vi "SMARP Software TCPIP - 100 - TS.vi"() -> (15 "error out":errorcluster={"status"=TRUE, "code"=2, "source"="FT_Open_Device_By_Index_2.vi<ERR>\nFT_DEVICE_NOT_FOUND"})   [LabVIEW 2015]
uses:
  Source code 64 bits/Global Cal Coefficients.vi
  Source code 64 bits/D_MON_Global_Save_Handling.vi
  Source code 64 bits/Global_Trig.vi
  <vilib>/Analysis/NI_AALPro.lvlib
  Source code 64 bits/Global Temp Coefficients.vi
  Source code 64 bits/Global line number.vi
  <vilib>/Utility/file.llb/Write To Spreadsheet File (DBL).vi
panel:
  out "Messages Sent":dbl
  out "String":string
  in  "Wait [ms]":u32=1000
  out "Length":i32
  out "Sending":bool
  in  "Transmission":bool caption="Blank Button"
  out "Scan rate [Hz]":dbl=100.0 format="%.1f"
  out "Total no. of scans":u64=20350
  out "Clear data loss":bool=TRUE
  out "No. of restarts":i16
  out "FT handle":u32=275386408
  in  "Number of pixels":u16=512
  out "Sensor temperature":dbl=29.5
  out "Status":bool=TRUE
  out "No. of scans without \ndata loss":u64=20350
  in  "Dark substraction":enum32{"3", "4"}(radio) caption="Substract dark"
  in  "Default dark spectrum":i32[](array[numeric])
  out "Data loss":bool
  out "Power saturated":bool
  out "Disk streaming enable":bool
  in  "Manuel save\nin datalog file":bool
  out "refnum out":refnum<file>
  out "Fitted Wavelength (nm) 2":dbl[][](array[numeric])=[[1595.5131620083362], [1595.5127751366058], [1595.5137326893469], [1595.5138830332794], [1595.5145223786622], [1595.514016514484], [1595.5136704516492], [1595.5140362639065], [1595.513886981301], [1595.5129422331306], [1595.5142763835854], [1595.5131991204937], [1595.5141702721774], [1595.5140596535118], [1595.513476018252], [1595.5130840632366], [1595.5133372352345], [1595.5143909134829], [1595.512547034042], [1595.5131347474842], [1595.5136018341527], [1595.5133635366617], [1595.5134215597598], [1595.5136216309304], [1595.5134388503177], [1595.514860425136], [1595.513637047946], [1595.5144108307254], [1595.5134006848923], [1595.5136540115332], [1595.5131151127853], [1595.5134841775725], [1595.5135582718326], [1595.51358873526], [1595.5144878935337], [1595.5133866872961], [1595.5135523397537], [1595.513956857277], [1595.5138624036094], [1595.513868537861], [1595.5141773781613], [1595.5139943040829], [1595.5140080784786], [1595.5136054910308], [1595.5132710852274], [1595.5136273367466], [1595.5134180231428], [1595.5137428127452], [1595.5134467206256], [1595.5124864680156], [1595.5133492708483], [1595.5138568551952], [1595.5139521788888], [1595.5129457857986], [1595.5134285012812], [1595.5132775616735], [1595.5138196678542], [1595.5134433791493], [1595.5131057080214], [1595.5135200395807], [1595.513512087234], [1595.512826806178], [1595.5147811740385], [1595.5136915283101], [1595.5137392114034], [1595.5125233078275], [1595.5143754672813], [1595.5137596894583], [1595.5138802243555], [1595.5136627382699], [1595.5128774801633], [1595.512992288448], [1595.5142936144803], [1595.5134010885834], [1595.5132554550344], [1595.5135961940969], [1595.5143572070504], [1595.5132616854469], [1595.5146787806843], [1595.5129005738843], [1595.5139568760248], [1595.5144654170813], [1595.5128774801633], [1595.5132012316803], [1595.5131706301513], [1595.5133248313573], [1595.5142833144234], [1595.5135630852683], [1595.5130317900264], [1595.513331497452], [1595.5139713766837], [1595.5138038514065], [1595.5139041777377], [1595.5136828192435], [1595.5133747159412], [1595.5136313106811], [1595.513910168194], [1595.5137736081301], [1595.5138395201484], [1595.5140244175132], [1595.5143887222805], [1595.513486738009], [1595.5122489667829], [1595.5122830246223], [1595.5131860770355], [1595.5135655715271], [1595.5132986015558], [1595.5129111513875], [1595.513646736944], [1595.512020396329], [1595.5133269476487], [1595.513158439359], [1595.5133154608318], [1595.513528581914], [1595.514587517312], [1595.513215473403], [1595.5133411671345], [1595.512850376517], [1595.513826716082], [1595.513113875053], [1595.5140448881584], [1595.5138417196122], [1595.5127217640932], [1595.5137354831563], [1595.5134230825417], [1595.5135733593886], [1595.2929746856532], [1595.51298986152], [1595.513021410847], [1595.5131545750744]] format="%.3f"
  out "Power Array":dbl[][](array[numeric]) format="%.2f"
  out "Dark spectrum":dbl[](array[numeric])
  in  "origin 2":cluster{"x":i16, "y":i16}
  out "new picture 2":picture
  in  "origin":cluster{"x":i16, "y":i16}={"x"=0, "y"=10}
  out "Fitted Wavelength (nm)":dbl[][](array[numeric]) format="%.4f"
  in  "Tab Control":T1(tab)
  out "Spectrum  Graph":cluster{dbl[], "Line spectrums":dbl[]}(graph)
  in  "Exposure time [usec]":dbl=10000.0 min=3.0 max=65535.0
  out "Wavelength Graph":T2(graph)={"f"=0.0, 0.0003333333333333333, "Rearranged array"=[]}
  out "Peak Frequency [Hz]":dbl[][](array[numeric]) format="%.2f"
  in  "FFT peak threshold [nm]":dbl=0.0005999999999999925 min=0.0 step=0.0001 format="%.5f"
  out "FFT Graph":T3(graph)
  in  "FFT calculation":enum32{"pix", "nm"}(radio)
  in  "Change datalog\nfile name":bool
  in  "Timed  data log":bool
  in  "Raw data collection":enum32{"3", "4"}(radio)
  in  "Disc streaming":enum32{"1", "2"}(radio)
  in  "X-Axis unit":enum32{"pix", "nm"}(radio)=enum."nm"
  in  "Measurement trig type":enum16{"Manuel", "Auto", "Continuous"}(ring)=enum."Continuous"
  in  "Max number \nof FBG's":u16=20 min=1
  in  "Threshold [%]":dbl=10.0
  in  "No. of frames to disc unified":i32=100
  in  "Trig frequency [Hz]":dbl=0.5 format="%.2f"
  in  "Circular Sample \nbuffer length":i32=3000
  in  "Wavelength/FFT graph buffer length":i32=3000
  out "Calibration coefficients":dbl[](array[numeric])=[1595.998689, -0.1387869764, -6.248194306e-05, -3.744159492e-09, 6.889567755e-13, -1.540737e-15] format="%.6e"
  out "Temperature coefficients":dbl[](array[numeric])=[-1.034429555e-06, 3.155140097e-05, -0.0001139713184, -0.004721861303] format="%.6e"
  in  "Change Disk stream\nfile name":bool
  in  "Neighbours in fit":i32=1
  in  "Change datalog\ntime interval":bool
  in  "Temperature \ncompensation":bool=TRUE
  in  "Exposure time\n[usec]":dbl=10000.0 min=3.0 max=65535.0
  in  "Fit Type":enum32{"Gauss", "COG", "COG DWA", "No fit"}(radio)=enum."COG DWA"
  in  "Max Scan rate [Hz]":i32=100 min=1 max=3000
  in  "No. of lines \nunified":u16=10 min=1 max=100 step=1
  in  "Offset (-250..250) mV":i32=-88
  in  "Path":path
  in  "Save Raw":bool
  in  "Save Wave":bool
  in  "Trig":bool
  in  "Exit":bool
  # "Ver 1.3"
  # "Peak no."
  # "Sample no."
  # "Peak no."
  # "FFT peak"
  # "Buffer setup"
  # "Camera setup"
  # "File setup"
  # "Interrogation setup"
  # "SW Trig setup"
  # "ID  information"
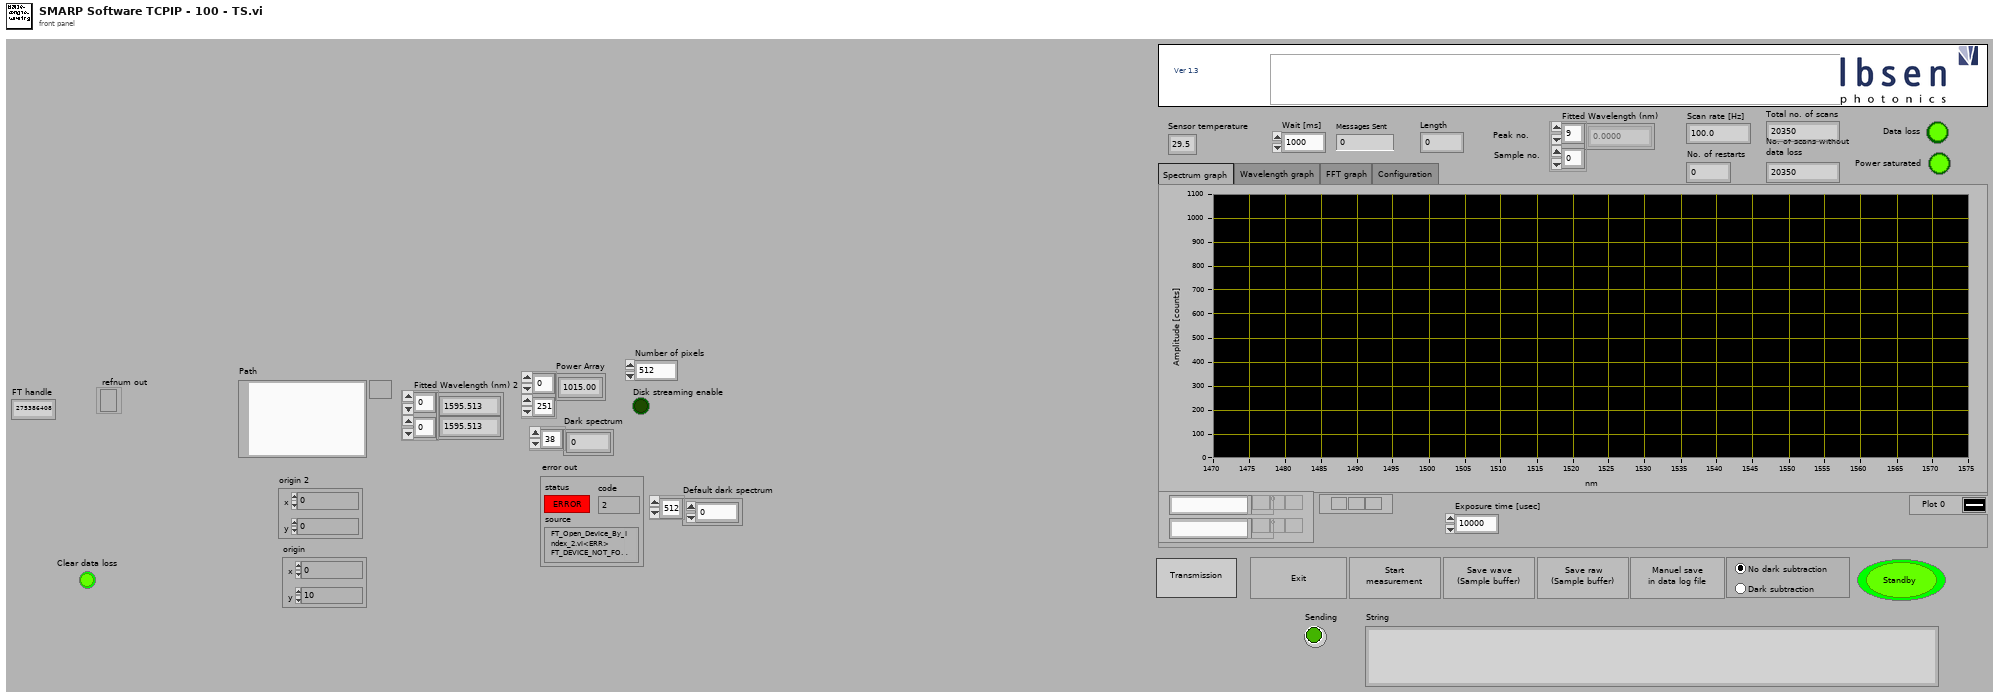
[diagram p1: front panel]
types:
  T1 = enum32{"Spectrum graph", "Wavelength graph", "FFT graph", "Configuration"}
  T2 = cluster{"f":dbl, dbl, "Rearranged array":dbl[][]}
  T3 = cluster{dbl, "df":dbl, "Amp Spectrum Mag (Vrms)":dbl[][]}
  T4 = enum16{"User-specified Font", "Application Font", "System Font", "Dialog Font"}
  T5 = cluster{"Font Name:":string, "Size":i16, "Strikeout?":bool, "Italic?":bool, "Underline?":bool, "Outline?":bool, "Shadow?":bool, "Bold?":bool}
  T6 = enum16{"open", "replace", "create", "open or create", "replace or create", "replace or create with confirmation"}
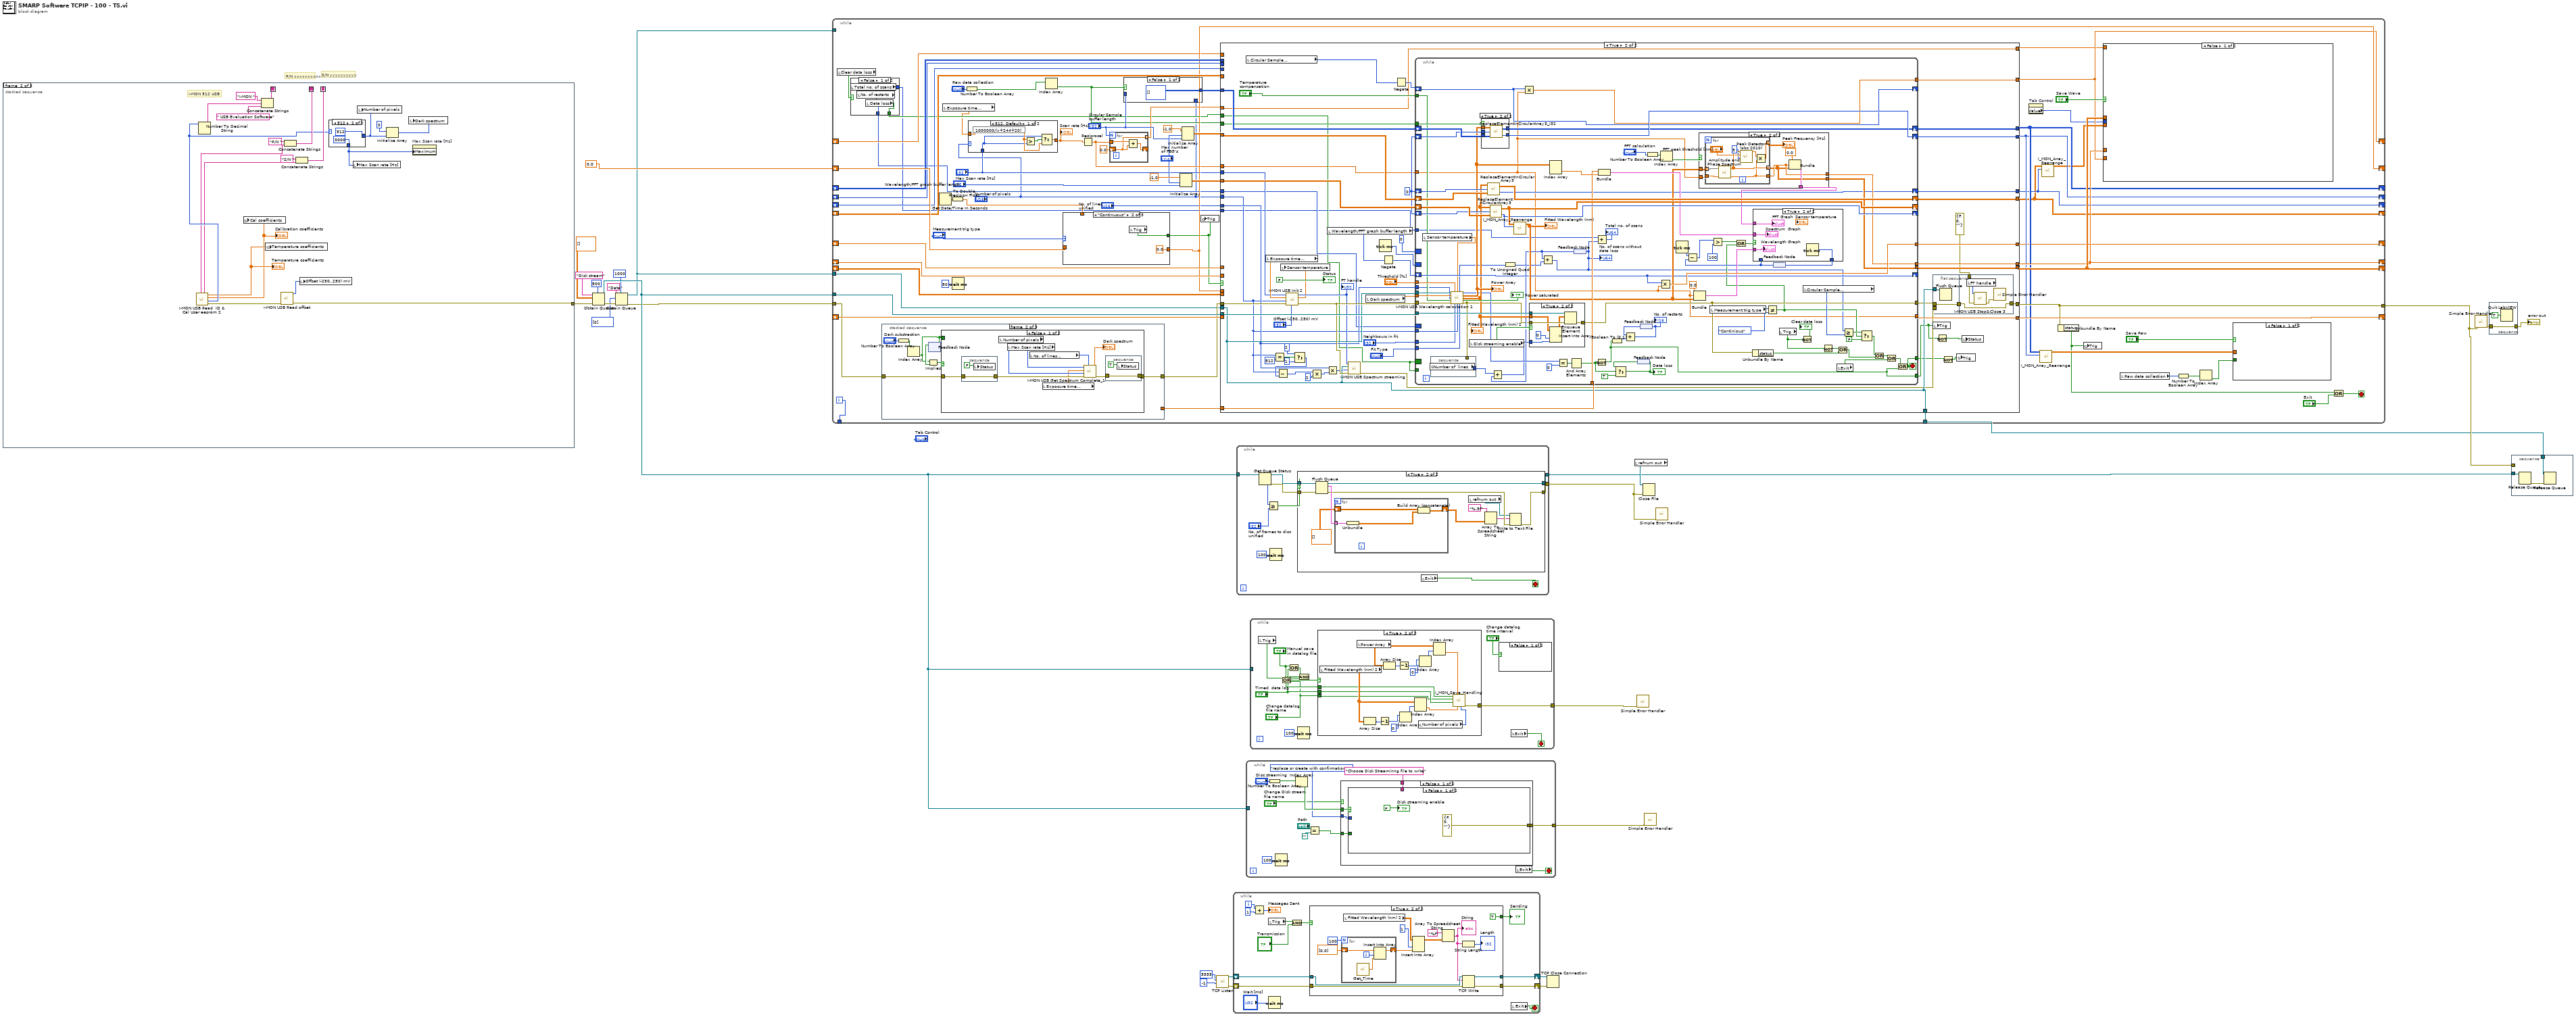
[diagram p0: block diagram]
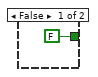
[diagram p2: hidden frame]
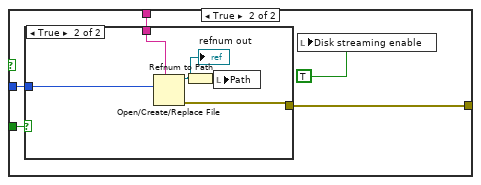
[diagram p3: hidden frame]
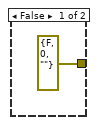
[diagram p4: hidden frame]
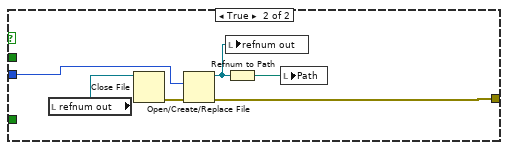
[diagram p5: hidden frame]
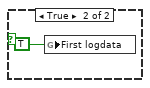
[diagram p6: hidden frame]
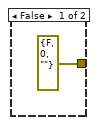
[diagram p7: hidden frame]
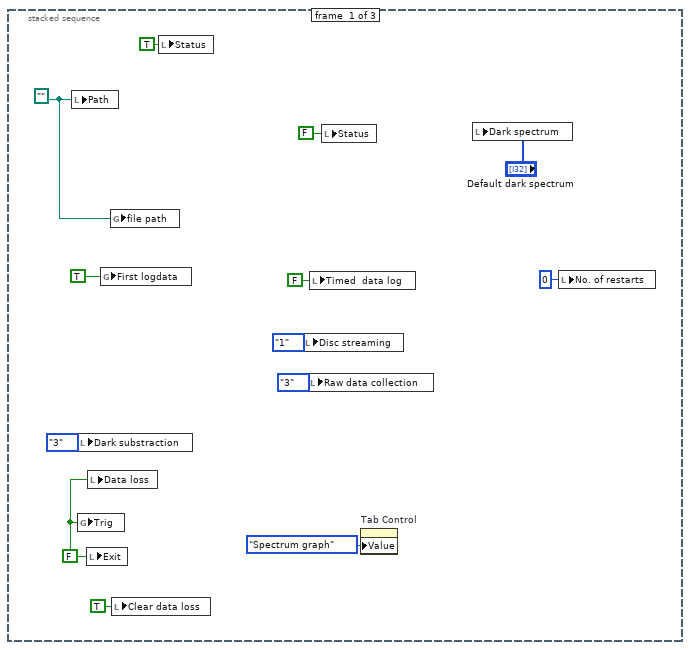
[diagram p8: hidden frame]
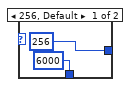
[diagram p9: hidden frame]
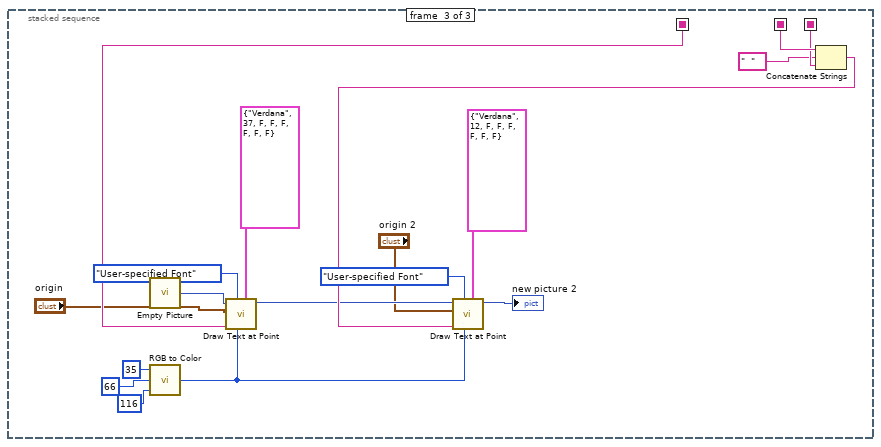
[diagram p10: hidden frame]
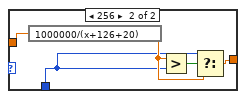
[diagram p12: hidden frame]
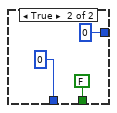
[diagram p13: hidden frame]
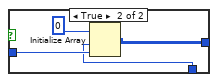
[diagram p14: hidden frame]
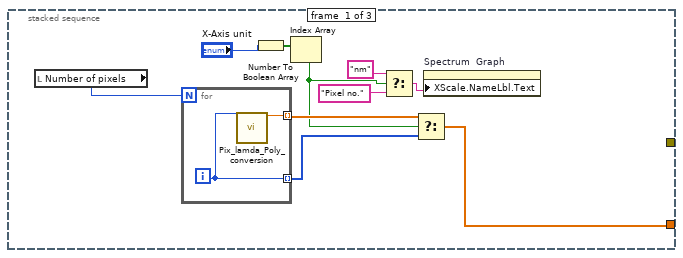
[diagram p15: hidden frame]
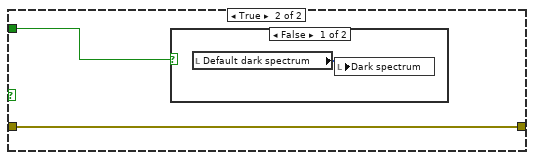
[diagram p16: hidden frame]
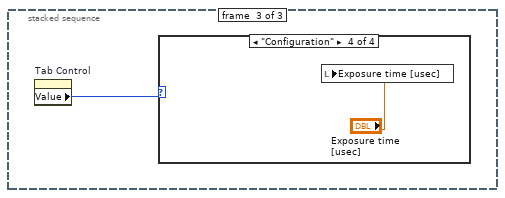
[diagram p18: hidden frame]
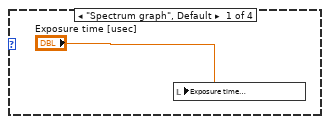
[diagram p19: hidden frame]
diagram:
  # "S/N yyyyyyyyyy"
  # "P/N xxxxxxxxxx"
  n1 = stacked-sequence {
    seq-local: [_ w60 _] -> [_ _ w71]
    seq-local: [_ w59 _] -> [_ _ w66]
    seq-local: [_ w57 _] -> [_ _ w76]
    tunnel: [_ w43 _] -> w22
    frame #0 {
      w29 = FALSE ("Exit")
      w37 = path ""
      n2 = local write "Path"(w37) -> ()
      n3 = local write "Dark substraction"(enum32{"3", "4"}."3" ("Dark substraction")) -> ()
      n4 = global write "Global_Trig.vi" "Trig"(w29) -> ()
      n5 = local write "Exit"(w29) -> ()
      n6 = local write "Data loss"(w29) -> ()
      n7 = global write "D_MON_Global_Save_Handling.vi" "First logdata"(TRUE ("First logdata")) -> ()
      n8 = global write "D_MON_Global_Save_Handling.vi" "file path"(w37) -> ()
      n9 = local write "Clear data loss"(TRUE ("Clear data loss")) -> ()
      n10 = local write "Status"(TRUE ("OK")) -> ()
      n11 = local write "Disc streaming"(enum32{"1", "2"}."1" ("Disk streaming")) -> ()
      n12 = local write "Raw data collection"(enum32{"3", "4"}."3" ("Raw data collection")) -> ()
      n13 = local write "Timed  data log"(FALSE ("Timed  datalog")) -> ()
      n14 = local write "Status"(FALSE ("Status")) -> ()
      n15 = property on="Tab Control" class="TabCtl (strict)"("Value"=T1."Spectrum graph" ("Tab Control")) -> ()  [unwired: 2 in, 2 out]
      n16 = local write "Dark spectrum"("Default dark spectrum") -> ()
      n17 = local write "No. of restarts"(i16 0 ("No. of restarts")) -> ()
    }
    frame #1 {
      # "I-MON 512 USB"
      n18 = call "I-MON USB Read  ID & Cal User eeprom 2.vi"() -> ("error out"=w44:errorcluster, "No. of pixels"=w51:i32, "Wave Cal coef"=w45:dbl[], "Temp Cal coef"=w46:dbl[], "Serial no."=w47:string, "Part no."=w49:string)  [unwired: 6 in]
      "Calibration coefficients" <- w45
      "Temperature coefficients" <- w46
      n19 = Number To Decimal String(number=w51) -> (decimal integer string=w52:string)  [unwired: 1 in]
      n20 = global write "Global Cal Coefficients.vi" "Cal coefficients"(w45) -> ()
      n21 = Concatenate Strings("I-MON " ("string"), w52, " USB Evaluation Software" ("text")) -> (w57:string)
      n22 = global write "Global Temp Coefficients.vi" "Temperature coefficients"(w46) -> ()
      n23 = call "I-MON USB Read offset.vi"("error in (no error)"=w44) -> ("error out"=w43:errorcluster, "Offset"=w42:i32)  [unwired: 9 in]
      n24 = Concatenate Strings("P/N " ("string"), w49) -> (w60:string)
      n25 = Concatenate Strings("S/N " ("string"), w47) -> (w59:string)
      n26 = local write "Offset (-250..250) mV"(w42) -> ()
      n27 = case shown="512" w51 {
        tunnel: [256 ("CCD Type") 512 ("CCD Type")] -> w55
        tunnel: [6000 ("CCD Type") 3000 ("CCD Type")] -> w41
        frame 256, Default {
        }
        frame 512 {
        }
      }
      n28 = local write "Max Scan rate [Hz]"(w41) -> ()
      n29 = local write "Number of pixels"(w55) -> ()
      n30 = Initialize Array(0, w55) -> (w54:i32[])
      n31 = local write "Dark spectrum"(w54) -> ()
      n32 = property on="Max Scan rate [Hz]" class="DigNum (strict)"("Maximum"=w41) -> ()  [unwired: 2 in, 2 out]
    }
    frame #2 {
      n33 = call "Empty Picture"() -> ("empty picture"=w82:picture)
      n34 = call <vilib>:"RGB to Color.vi"("B"=u8 116, "G"=u8 66, "R"=u8 35) -> ("Color"=w73:u32)
      n35 = call <vilib>:"Draw Text at Point.vi"("[user-specified font]"=T5 {"Font Name:"="Verdana", "Size"=37, "Strikeout?"=FALSE, "Italic?"=FALSE, "Underline?"=FALSE, "Outline?"=FALSE, "Shadow?"=FALSE, "Bold?"=FALSE}, "text color(black)"=w73, "desired font(Application)"=T4."User-specified Font", "text"=w76, "origin"="origin", "picture"=w82) -> ("new picture"=w68:picture)  [unwired: 4 in, 1 out]
      n36 = Concatenate Strings(w71, "  " ("string"), w66) -> (w70:string)
      n37 = call <vilib>:"Draw Text at Point.vi"("[user-specified font]"=T5 {"Font Name:"="Verdana", "Size"=12, "Strikeout?"=FALSE, "Italic?"=FALSE, "Underline?"=FALSE, "Outline?"=FALSE, "Shadow?"=FALSE, "Bold?"=FALSE}, "text color(black)"=w73, "desired font(Application)"=T4."User-specified Font", "text"=w70, "origin"="origin 2", "picture"=w68) -> ("new picture"=→"new picture 2":picture)  [unwired: 4 in, 1 out]
    }
  }
  n38 = Obtain Queue(max queue size (-1, unlimited)=500, name (unnamed)="Disk stream", element data type=dbl[][] [], error in (no error)=w22) -> (queue out=w18:refnum<queue>, error out=w16:errorcluster)  [unwired: 1 in, 1 out]
  n39 = Obtain Queue(max queue size (-1, unlimited)=1000, name (unnamed)="Data", element data type=u8[] [0], error in (no error)=w16) -> (queue out=w11:refnum<queue>, error out=w15:errorcluster)  [unwired: 1 in, 1 out]
  n40 = while {
    tunnel: [w134] -> w23
    shift-right: [w117] -> _
    shift-left: 0.0 ("seconds since 1Jan1904") -> [w147]
    shift-right: [w143] -> _
    shift-left: _ -> [w144]
    shift-right: [w142] -> _
    shift-left: _ -> [w140]
    shift-right: [w139] -> _
    shift-left: _ -> [w141]
    tunnel: w15 -> [w109]
    shift-right: [w121] -> _
    shift-left: _ -> [w129]
    shift-right: [w122] -> _
    shift-left: _ -> [w128]
    shift-right: [w123] -> _
    shift-left: _ -> [w125]
    shift-right: [w124] -> _
    shift-left: _ -> [w126]
    shift-right: [w118] -> _
    shift-left: _ -> [w119]
    shift-right: [w115] -> _
    shift-left: _ -> [w116]
    tunnel: w18 -> [w114]
    tunnel: w11 -> [_]
    tunnel: w11 -> [w106]
    tunnel: [w105] -> w10
    tunnel: [w103] -> _
    i -> [w103]
    stop <- w149 stop-if-true
    n41 = local read "Clear data loss"() -> (w91:bool)
    n42 = case shown="False" w91 {
      tunnel: [w163 i16 0] -> w93
      tunnel: [w162 FALSE ("Data loss")] -> w92
      tunnel: [w161 u64 0 ("Total no. of scans")] -> w90
      frame False {
        n43 = local read "Total no. of scans"() -> (w161:u64)
        n44 = local read "No. of restarts"() -> (w163:i16)
        n45 = local read "Data loss"() -> (w162:bool)
      }
      frame True {
      }
    }
    n46 = stacked-sequence {
      tunnel: [w182 _ _] -> w112
      tunnel: w109 -> [_ w193 _]
      tunnel: [_ w192 _] -> w108
      frame #0 {
        n47 = local read "Number of pixels"() -> (w175:u16)
        n48 = for {
          N: w175 -> [_]
          tunnel: [w186] -> w183 mode=indexing
          tunnel: [w185] -> w184 mode=indexing
          i -> [w185]
          n49 = call "Pix_lamda_Poly_conversion.vi"("Pixels"=w185) -> ("Lamda(nm)"=w186:dbl)  [unwired: 8 in, 6 out]
        }
        n50 = Number To Boolean Array(number="X-Axis unit") -> (Boolean array=w181:bool[])
        n51 = Index Array(array=w181) -> (element=w176:bool)  [unwired: 1 in]
        n52 = Select(t="nm", s=w176, f="Pixel no.") -> (s? t:f=w179:string)
        n53 = Select(t=w183, s=w176, f=w184) -> (s? t:f=w182:dbl[])
        n54 = property on="Spectrum  Graph" class="XYGraph (strict)"("XScale.NameLbl.Text"=w179) -> ()  [unwired: 2 in, 2 out]
      }
      frame #1 {
        n55 = Number To Boolean Array(number="Dark substraction") -> (Boolean array=w189:bool[])
        n56 = Index Array(array=w189) -> (element=w187:bool)  [unwired: 1 in]
        n57 = feedback-in #1(w187) -> ()
        n58 = feedback #1() -> (w191:bool)  [unwired: 1 in]
        n59 = Implies(1:w191, 2:w187) -> (0:w190:bool)
        n60 = case shown="False" w190 {
          tunnel: w193 -> [w202 w208]
          tunnel: [w200 w208] -> w192
          tunnel: w187 -> [_ w207]
          frame False {
            n61 = stacked-sequence {
              tunnel: w202 -> [w205]
              tunnel: [w205] -> w201
              frame #0 {
                n62 = local write "Status"(FALSE ("Status")) -> ()
              }
            }
            n63 = local read "Number of pixels"() -> (w195:u16)
            n64 = local read "Max Scan rate [Hz]"() -> (w196:i32)
            n65 = local read "No. of lines \nunified"() -> (w197:u16)
            n66 = local read "Exposure time\n[usec]"() -> (w194:dbl)
            n67 = call "I-MON USB Get Spectrum Complete_1.vi"("Number of avg spectrums"=w197, "error in (no error)"=w201, "No of pixels"=w195, "Integration time [us]"=w194, "Sample frequency"=w196) -> ("error out"=w198:errorcluster, "Line spectrums"=→"Dark spectrum":dbl[])  [unwired: 5 in]
            n68 = stacked-sequence {
              tunnel: w198 -> [w203]
              tunnel: [w203] -> w200
              frame #0 {
                n69 = local write "Status"(TRUE ("Status")) -> ()
              }
            }
          }
          frame True {
            n70 = case shown="False" w207 {
              frame False {
                n71 = local read "Default dark spectrum"() -> (w209:i32[])
                n72 = local write "Dark spectrum"(w209) -> ()
              }
              frame True {
              }
            }
          }
        }
      }
      frame #2 {
        n73 = property on="Tab Control" class="TabCtl (strict)"() -> ("Value"=w210:T1)  [unwired: 2 in, 2 out]
        n74 = case shown="\"Configuration\"" w210 {
          frame "Spectrum graph", Default {
            n75 = local write "Exposure time\n[usec]"("Exposure time [usec]") -> ()
          }
          frame "Wavelength graph" {
          }
          frame "FFT graph" {
          }
          frame "Configuration" {
            n76 = local write "Exposure time [usec]"("Exposure time\n[usec]") -> ()
          }
        }
      }
    }
    n77 = Get Date/Time In Seconds() -> (seconds since 1Jan1904=w138:timestamp)
    n78 = local read "Exposure time\n[usec]"() -> (w86:dbl)
    n79 = To Double Precision Float(number=w138) -> (double precision float=w148:dbl)
    n80 = Wait (ms)(milliseconds to wait=u32 50) -> ()  [unwired: 1 out]
    n81 = Number To Boolean Array(number="Raw data collection") -> (Boolean array=w110:bool[])
    n82 = case shown="512, Default" "Number of pixels" {
      tunnel: w86 -> [w153 w160]
      tunnel: [w152 w157] -> w83
      tunnel: "Max Scan rate [Hz]" -> [w151 w156]
      frame 512, Default {
        n83 = expression code="1000000/(x+244+20)"(w153) -> (w154:dbl)
        n84 = Greater?(x=w154, y=w151) -> (0:w155:bool)
        n85 = Select(t=w151, s=w155, f=w154) -> (s? t:f=w152:dbl)
      }
      frame 256 {
        n86 = expression code="1000000/(x+126+20)"(w160) -> (w158:dbl)
        n87 = Greater?(x=w158, y=w156) -> (0:w159:bool)
        n88 = Select(t=w156, s=w159, f=w158) -> (s? t:f=w157:dbl)
      }
    }
    "Scan rate [Hz]" <- w83
    n89 = Index Array(array=w110) -> (element=w89:bool)  [unwired: 1 in]
    n90 = case shown="\"Continuous\"" "Measurement trig type" {
      tunnel: w148 -> [_ _ w285]
      tunnel: [0.0 ("seconds since 1Jan1904") 0.0 ("seconds since 1Jan1904") w283] -> w117
      tunnel: w147 -> [_ _ w278]
      tunnel: ["Trig" w277 w280] -> w104
      frame "Manuel", Default {
      }
      frame "Continuous" {
        n91 = local read "Trig"() -> (w277:bool)
      }
      frame "Auto" {
        n92 = Reciprocal(x="Trig frequency [Hz]") -> (1/x=w281:dbl)
        n93 = Add(x=w278, y=w281) -> (x+y=w279:dbl)
        n94 = Greater Or Equal?(x=w285, y=w279) -> (x >= y?=w284:bool)
        n95 = case shown="False" w284 {
          tunnel: [w287 w290] -> w283
          tunnel: w278 -> [w287 _]
          tunnel: [w286 w288] -> w280
          frame False {
            w286 = FALSE
            n96 = local write "Trig"(w286) -> ()
          }
          frame True {
            w288 = TRUE
            n97 = Get Date/Time In Seconds() -> (seconds since 1Jan1904=w289:timestamp)
            n98 = local write "Trig"(w288) -> ()
            n99 = To Double Precision Float(number=w289) -> (double precision float=w290:dbl)
          }
        }
      }
    }
    n100 = Reciprocal(x=w83) -> (1/x=w87:dbl)
    n101 = for {
      N: "Circular Sample \nbuffer length" -> [_]
      tunnel: w87 -> [w168]
      shift-right: [w169] -> _
      shift-left: 0.0 -> [w167]
      tunnel: [w167] -> w95 mode=indexing
      n102 = Add(x=w168, y=w167) -> (x+y=w169:dbl)
    }
    n103 = case shown="False" w89 {
      tunnel: "Circular Sample \nbuffer length" -> [_ w174]
      tunnel: [i32[][] [] ("f") w172] -> w107
      tunnel: "Number of pixels" -> [_ w171]
      frame False {
      }
      frame True {
        n104 = Initialize Array(u16 0, w171, w174) -> (w172:u16[][])
      }
    }
    n105 = Initialize Array(-1.0 ("element"), "Max number \nof FBG's", "Wavelength/FFT graph buffer length") -> (w131:dbl[][])
    n106 = Initialize Array(-1.0 ("element"), "Max number \nof FBG's", "Circular Sample \nbuffer length") -> (w135:dbl[][])
    n107 = global write "Global_Trig.vi" "Trig"(w104) -> ()
    n108 = case shown="True" w104 {
      tunnel: [w292 w341] -> w134
      tunnel: w117 -> [_ _]
      tunnel: [w302 w363] -> w143
      tunnel: w144 -> [w302 _]
      tunnel: [w300 w362] -> w142
      tunnel: [w301 w360] -> w139
      tunnel: w141 -> [w301 _]
      tunnel: w140 -> [w300 _]
      tunnel: w108 -> [w292 w361]
      tunnel: w135 -> [_ w359]
      tunnel: w131 -> [_ w358]
      tunnel: [w299 w355] -> w121
      tunnel: [w298 w354] -> w122
      tunnel: w129 -> [w299 _]
      tunnel: w128 -> [w298 _]
      tunnel: w107 -> [_ w353]
      tunnel: [w297 w352] -> w124
      tunnel: [w296 w351] -> w123
      tunnel: w126 -> [w297 _]
      tunnel: w125 -> [w296 _]
      tunnel: [w295 w350] -> w118
      tunnel: w119 -> [w295 _]
      tunnel: [w294 w348] -> w115
      tunnel: w116 -> [w294 _]
      tunnel: w89 -> [_ w346]
      tunnel: w114 -> [_ w345]
      tunnel: w112 -> [_ w344]
      tunnel: w106 -> [w293 w333]
      tunnel: [w293 w333] -> w105
      tunnel: "Max Scan rate [Hz]" -> [_ w327]
      tunnel: "No. of lines \nunified" -> [_ w314]
      tunnel: "Number of pixels" -> [_ w313]
      tunnel: w95 -> [w291 w311]
      tunnel: [w291 w311] -> w94
      tunnel: w93 -> [_ w309]
      tunnel: w92 -> [_ w308]
      tunnel: w90 -> [_ w305]
      tunnel: w87 -> [_ w303]
      frame False {
      }
      frame True {
        w338 = u32 0
        n109 = local read "Circular Sample \nbuffer length"() -> (w336:i32)
        n110 = local read "Exposure time\n[usec]"() -> (w328:dbl)
        n111 = Equal?(x=w313, y=u16 512) -> (x = y?=w321:bool)
        n112 = call "I-MON USB Init 2.vi"("Offset (-250..250) mV"="Offset (-250..250) mV", "error in (no error)"=w361, "No of pixels"=w313, "Integration time [us]"=w328, "Max Sample frequency"=w327) -> ("error out"=w340:errorcluster, "Temperature"=w312:dbl, "Handle"=w323:u32)  [unwired: 4 in]
        "FT handle" <- w323
        n113 = local write "Sensor temperature"(w312) -> ()
        n114 = Select(t=u16 2 ("y"), s=w321, f=u16 1) -> (s? t:f=w317:u16)
        n115 = Subtract(x=w313, y=w317) -> (x-y=w316:u16)
        n116 = Multiply(x=w316, y=2) -> (x*y=w324:i32)
        n117 = Multiply(x=w314, y=w324) -> (x*y=w318:i32)
        n118 = local read "Wavelength/FFT graph buffer length"() -> (w337:i32)
        n119 = call "I-MON USB Spectrum streaming.vi"("error in (no error)"=w340, "Bytes To Read"=w318, "queue in"=w333, "Handle"=w323) -> ("error out"=w331:errorcluster)  [unwired: 7 in]
        n120 = local read "Dark spectrum"() -> (w343:dbl[])
        n121 = Tick Count (ms)() -> (millisecond timer value=w342:u32)
        n122 = Negate(x=w337) -> (-x=w357:i32)
        n123 = Negate(x=w336) -> (-x=w349:i32)
        n124 = while {
          tunnel: w340 -> [w458]
          tunnel: [w429] -> w332
          tunnel: [w414] -> w363
          tunnel: [w415] -> w362
          tunnel: "Fit Type" -> [w399]
          tunnel: [w370] -> w360
          shift-right: [w409] -> w354
          shift-left: w338 -> [w455]
          shift-right: [w453] -> w355
          shift-left: w359 -> [w454]
          shift-right: [w437] -> _
          shift-left: w358 -> [w456]
          shift-right: [w436] -> _
          shift-left: w338 -> [w452]
          shift-right: [w412] -> _
          shift-left: w357 -> [w412]
          shift-right: [w438] -> w352
          shift-left: w353 -> [w444]
          shift-right: [w443] -> w351
          shift-left: w338 -> [w442]
          tunnel: [w441] -> w350
          shift-right: [w411] -> _
          shift-left: w349 -> [w411]
          tunnel: [w440] -> w348
          tunnel: "Threshold [%]" -> [w439]
          tunnel: w303 -> [w370]
          border: w308 -> [_]
          tunnel: w346 -> [w435]
          tunnel: w345 -> [w434]
          tunnel: w344 -> [w432]
          tunnel: w343 -> [w405]
          tunnel: w333 -> [w406]
          border: w342 -> [_]
          tunnel: "Temperature \ncompensation" -> [w404]
          tunnel: w313 -> [w398]
          tunnel: "Neighbours in fit" -> [w397]
          tunnel: w314 -> [w396]
          tunnel: w308 -> [_]
          border: u64 0 -> [_]
          tunnel: [w387] -> w310
          border: w309 -> [_]
          tunnel: [w382] -> w307
          tunnel: w305 -> [w378]
          stop <- w382 stop-if-true
          n125 = local read "Sensor temperature"() -> (w403:dbl)
          n126 = call "I-MON USB Wavelength calculation 1.vi"("queue"=w406, "Threshold\n[%]"=w439, "PCB temperature"=w403, "Dark meas"=w405, "No. of spectrums"=w396, "Temp. compensation"=w404, "error in (no error)"=w458, "Neighbours in fit"=w397, "Number of pixels"=w398, "Fit Type"=w399) -> ("No. of line scans"=w391:i32, "Delimiter"=w394:u16[], "Line spectrums"=w401:dbl[][], "Center pixels (0 indexeret)"=w400:dbl[][], "Power saturated"=→"Power saturated":bool, "error out"=w372:errorcluster)
          "Power Array" <- w401
          "Fitted Wavelength (nm) 2" <- w400
          n127 = stacked-sequence {
            tunnel: [w459] -> w375
            tunnel: w372 -> [_]
            frame #0 {
              n128 = global read "Global line number.vi" "Number of  lines"() -> (w459:i32[])
            }
          }
          n129 = local read "Disk streaming enable"() -> (w433:bool)
          n130 = case shown="True" w435 {
            tunnel: w401 -> [_ w497]
            tunnel: w444 -> [w492 w496]
            tunnel: [w491 w495] -> w443
            tunnel: w442 -> [w491 w494]
            tunnel: [w492 w493] -> w438
            frame False {
            }
            frame True {
              n131 = call "ReplaceElementInCircularArray3_I32.vi"("Initial Array - Before Element Inserted"=w496, "Original Element's Index"=w494, "Inserted Array"=w497) -> ("New Element Index \nfor Circular Array"=w495:u32, "Output Circular Array - After Inserting Element"=w493:i32[][])
            }
          }
          n132 = call "ReplaceElementInCircularArray3.vi"("Initial Array - Before Element Inserted"=w454, "Original Element's Index"=w455, "Inserted Array"=w400) -> ("New Element Index \nfor Circular Array"=w409:u32, "Output Circular Array - After Inserting Element"=w453:dbl[][])
          n133 = call "ReplaceElementInCircularArray3.vi"("Initial Array - Before Element Inserted"=w456, "Original Element's Index"=w452, "Inserted Array"=w400) -> ("New Element Index \nfor Circular Array"=w436:u32, "Output Circular Array - After Inserting Element"=w437:dbl[][])
          n134 = To Unsigned Quad Integer(1:w391) -> (0:w377:u64)
          n135 = call "I_MON_Array_Rearrange.vi"("index"=w436, "Initial Array"=w437) -> ("Rearranged array"=w416:dbl[][])  [unwired: 9 in]
          "Fitted Wavelength (nm)" <- w416
          n136 = Multiply(x=w411, y=w370) -> (x*y=w440:dbl)
          n137 = Index Array(array=w401) -> (element=w431:dbl[])  [unwired: 2 in]
          n138 = Equal?(x=w394, y=u16 0 ("Delimiter")) -> (x = y?=w395:bool[])
          n139 = And Array Elements(Boolean array=w395) -> (logical AND=w390:bool)
          n140 = feedback #2() -> (w373:u64)
          n141 = Add(x=w375, y=w373) -> (x+y=w374:u64[])
          n142 = case shown="True" w433 {
            tunnel: w434 -> [_ w490]
            tunnel: w400 -> [_ w486]
            tunnel: w372 -> [w483 w489]
            tunnel: [w483 w488] -> w429
            tunnel: w374 -> [_ w484]
            frame False {
            }
            frame True {
              n143 = Insert Into Array(array=w486, index (col)=0 ("disabled index (col)"), new element=w484) -> (w485:dbl[][])  [unwired: 1 in]
              n144 = Enqueue Element(queue=w490, element=w485, error in (no error)=w489) -> (error out=w488:errorcluster)  [unwired: 1 in, 2 out]
            }
          }
          n145 = Add(x=w373, y=w377) -> (x+y=w376:u64)
          "No. of scans without \ndata loss" <- w376
          n146 = feedback-in #2(w376) -> ()
          n147 = Not(x=w390) -> (.not. x?=w387:bool)
          n148 = Add(x=w378, y=w376) -> (x+y=→"Total no. of scans":u64)
          n149 = Bundle(w432, "Line spectrums"=w431) -> (w421:cluster{dbl[], "Line spectrums":dbl[]})  [unwired: 1 in]
          n150 = Boolean To (0,1)(Boolean=w387) -> (0, 1=w389:i16)
          n151 = feedback #3() -> (w384:bool)
          n152 = Select(t=w384, s=w390, f=TRUE ("Status")) -> (s? t:f=w386:bool)
          "Data loss" <- w386
          n153 = feedback-in #3(w386) -> ()
          n154 = feedback #4() -> (w388:i16)
          n155 = Add(x=w388, y=w389) -> (x+y=w385:i16)
          "No. of restarts" <- w385
          n156 = feedback-in #4(w385) -> ()
          n157 = Number To Boolean Array(number="FFT calculation") -> (Boolean array=w419:bool[])
          n158 = Multiply(x=w412, y=w370) -> (x*y=w441:dbl)
          n159 = Index Array(array=w419) -> (element=w418:bool)  [unwired: 1 in]
          n160 = Tick Count (ms)() -> (millisecond timer value=w425:u32)
          n161 = Bundle("f"=0.0, w370, "Rearranged array"=w416) -> (w426:T2)  [unwired: 1 in]
          n162 = case shown="True" w418 {
            tunnel: w416 -> [_ w467]
            tunnel: w370 -> [_ w466]
            tunnel: [T3 {0.0, "df"=0.0, "Amp Spectrum Mag (Vrms)"=[]} w465] -> w420
            tunnel: [0.0 ("df") w464] -> w415
            tunnel: [dbl[][] [] ("Amp Spectrum Mag (Vrms)") w463] -> w414
            frame False {
            }
            frame True {
              n163 = for {
                tunnel: [w475] -> w463 mode=indexing
                tunnel: [w474] -> w464
                tunnel: w466 -> [w477]
                tunnel: w467 -> [w476] mode=indexing
                tunnel: [w473] -> w469 mode=indexing
                n164 = call <vilib>:"Amplitude and Phase Spectrum.vi"("dt"=w477, "Signal (V)"=w476) -> ("df"=w474:dbl, "Amp Spectrum Mag (Vrms)"=w475:dbl[])  [unwired: 1 in, 1 out]
                n165 = call <vilib>:"Peak Detector (obs 2010).vi"("width"=5, "threshold"="FFT peak threshold [nm]", "X"=w475) -> ("Locations"=w470:dbl[])  [unwired: 4 in, 4 out]
                n166 = Multiply(x=w470, y=w474) -> (x*y=w473:dbl[])
              }
              "Peak Frequency [Hz]" <- w469
              n167 = Bundle(0.0, "df"=w464, "Amp Spectrum Mag (Vrms)"=w463) -> (w465:T3)  [unwired: 1 in]
            }
          }
          n168 = local read "Measurement trig type"() -> (w449:enum16{"Manuel", "Auto", "Continuous"})
          n169 = Unbundle By Name(w429) -> ("status"=w371:bool)
          n170 = Not Equal?(x=w449, y=enum16{"Manuel", "Auto", "Continious"}."Continious" ("Trig type")) -> (x != y?=w407:bool)
          n171 = feedback #5() -> (w422:u32)
          n172 = Subtract(x=w425, y=w422) -> (x-y=w424:u32)
          n173 = Greater?(x=w424, y=u32 100) -> (0:w428:bool)
          n174 = Or(x=w428, y=w407) -> (x .or. y?=w408:bool)
          n175 = case shown="True" w408 {
            tunnel: w426 -> [_ w482]
            tunnel: [w478 w481] -> w423
            tunnel: w422 -> [w478 _]
            tunnel: w421 -> [_ w480]
            tunnel: w420 -> [_ w479]
            frame False {
            }
            frame True {
              n176 = Tick Count (ms)() -> (millisecond timer value=w481:u32)
              "Wavelength Graph" <- w482
              "Spectrum  Graph" <- w480
              "FFT Graph" <- w479
            }
          }
          n177 = feedback-in #5(w423) -> ()
          n178 = local read "Trig"() -> (w381:bool)
          n179 = Not(x=w381) -> (.not. x?=→"Clear data loss":bool)
          n180 = local read "Circular Sample \nbuffer length"() -> (w410:i32)
          n181 = Not(x=w381) -> (.not. x?=w457:bool)
          n182 = local read "Exit"() -> (w413:bool)
          n183 = Or(x=w457, y=w371) -> (x .or. y?=w450:bool)
          n184 = Greater Or Equal?(x=w376, y=w410) -> (x >= y?=w447:bool)
          n185 = Select(t=w447, s=w407, f=FALSE) -> (s? t:f=w446:bool)
          n186 = Or(x=w446, y=w450) -> (x .or. y?=w430:bool)
          n187 = Or(x=w430, y=w413) -> (x .or. y?=w383:bool)
          n188 = Or(x=w383, y=w387) -> (x .or. y?=w382:bool)
        }
        n189 = flat-sequence {
          tunnel: w332 -> [w365]
          tunnel: [w365] -> w334
          tunnel: w333 -> [w364]
          tunnel: w331 -> [_]
          tunnel: [w369] -> w341
          tunnel: errorcluster {"status"=FALSE, "code"=0, "source"=""} ("error out") -> [w368]
          tunnel: w334 -> [w369]
          frame #0 {
            n190 = Flush Queue(queue=w364) -> ()  [unwired: 1 in, 3 out]
          }
          frame #1 {
            n191 = local read "FT handle"() -> (w367:u32)
            n192 = call "I-MON USB Stop&Close 3.vi"("error in (no error)"=w368, "Handle"=w367) -> ("error out"=w366:errorcluster)  [unwired: 9 in]
            n193 = call <vilib>:"Simple Error Handler.vi"("error in (no error)"=w366) -> ()  [unwired: 4 in, 5 out]
          }
        }
        n194 = local write "Trig"(w310) -> ()
        n195 = Not(x=w310) -> (.not. x?=w356:bool)
        n196 = Not(x=w307) -> (.not. x?=w306:bool)
        n197 = global write "Global_Trig.vi" "Trig"(w306) -> ()
        n198 = local write "Status"(w356) -> ()
        "Status" <- FALSE ("Status")
      }
    }
    n199 = property on="Tab Control" class="TabCtl (strict)"() -> ("Value"=w113:T1)  [unwired: 2 in, 2 out]
    n200 = call "I_MON_Array_Rearrange.vi"("index"=w123, "Initial Array"=w124) -> ("Rearranged array"=w127:dbl[][])  [unwired: 9 in]
    n201 = call "I_MON_Array_Rearrange.vi"("index"=w122, "Initial Array"=w121) -> ("Rearranged array"=w120:dbl[][])  [unwired: 9 in]
    n202 = Unbundle By Name(w134) -> ("status"=w88:bool)
    n203 = global write "Global_Trig.vi" "Trig"(w88) -> ()
    n204 = case shown="False" "Save Wave" {
      tunnel: w143 -> [_ w230]
      tunnel: w120 -> [_ w229]
      tunnel: w113 -> [_ w223]
      tunnel: w142 -> [_ w224]
      tunnel: w115 -> [_ _]
      tunnel: w94 -> [_ w219]
      frame False {
      }
      frame True {
        n205 = case shown="\"Wavelength graph\", Default" w223 {
          tunnel: w230 -> [_ _ _ w260]
          tunnel: [w251 w255 w259 w260] -> w228
          tunnel: w229 -> [w251 w255 w259 _]
          tunnel: ["Time [sec]\t" ("format (%.3f)") "Time [sec]\t" ("format (%.3f)") "Time [sec]\t" ("format (%.3f)") "Frequency [Hz]\t" ("format (%.3f)")] -> w227
          tunnel: ["Wavelength " ("format (%.3f)") "Wavelength " ("format (%.3f)") "Wavelength " ("format (%.3f)") "Wavelength " ("format (%.3f)")] -> w226
          tunnel: ["[nm]\t" ("string") "[nm]\t" ("string") "[nm]\t" ("string") "[nm RMS]\t" ("string")] -> w225
          frame "Wavelength graph", Default {
          }
          frame "Configuration" {
          }
          frame "Spectrum graph" {
          }
          frame "FFT graph" {
          }
        }
        n206 = Array Size(array=w228) -> (size(s)=w240:i32[])
        n207 = Index Array(array=w240, index=1) -> (element=w243:i32)
        n208 = for {
          N: w243 -> [_]
          tunnel: w224 -> [w272]
          shift-right: [w273] -> _
          shift-left: 0.0 -> [w271]
          tunnel: [w271] -> w221 mode=indexing
          n209 = Add(x=w271, y=w272) -> (x+y=w273:dbl)
        }
        n210 = case shown="\"FFT graph\"" w223 {
          tunnel: w219 -> [w244 w245 _ w247]
          tunnel: [w244 w245 w246 w247] -> w222
          tunnel: w221 -> [_ _ w246 _]
          frame "Spectrum graph", Default {
          }
          frame "Wavelength graph" {
          }
          frame "FFT graph" {
          }
          frame "Configuration" {
          }
        }
        n211 = Build Array (concatenate)(w222, w228) -> (w232:dbl[][])
        n212 = Transpose 2D Array(2D array=w232) -> (transposed array=w231:dbl[][])
        n213 = Index Array(array=w240, index=0) -> (element=w238:i32)
        n214 = for {
          N: w238 -> [_]
          shift-right: [w270] -> w236
          shift-left: "" ("format (%.3f)") -> [w265]
          tunnel: w226 -> [w264]
          tunnel: w225 -> [w268]
          i -> [w266]
          n215 = Increment(x=w266) -> (x+1=w267:i32)
          n216 = Number To Decimal String(number=w267) -> (decimal integer string=w269:string)  [unwired: 1 in]
          n217 = Concatenate Strings(w265, w264, w269, w268) -> (w270:string)
        }
        n218 = Array To Spreadsheet String(array=w231, 3:"%.7f" ("format (%.3f)")) -> (spreadsheet string=w234:string)  [unwired: 1 in]
        n219 = Concatenate Strings(w227, w236, "\r\n", w234) -> (w233:string)
        n220 = call <vilib>:"Write Characters To File.vi"("character string"=w233) -> ()  [unwired: 4 in, 1 out]
      }
    }
    n221 = local read "Raw data collection"() -> (w101:enum32{"3", "4"})
    n222 = Number To Boolean Array(number=w101) -> (Boolean array=w102:bool[])
    n223 = Index Array(array=w102) -> (element=w100:bool)  [unwired: 1 in]
    n224 = case shown="False" "Save Raw" {
      tunnel: w127 -> [_ w214]
      tunnel: w100 -> [_ w213]
      frame False {
      }
      frame True {
        n225 = case shown="False" w213 {
          tunnel: w214 -> [_ w218]
          frame False {
            n226 = One Button Dialog(message="Raw data collection is disabled !") -> ()  [unwired: 1 in, 1 out]
          }
          frame True {
            n227 = call-poly <vilib>:"Write To Spreadsheet File.vi"("transpose? (no:F)"=TRUE, "format (%.3f)"="%.5d" ("format string"), "2D data"=w218) -> ()  [unwired: 5 in, 1 out]
          }
        }
      }
    }
    n228 = Or(x=w88, y="Exit") -> (x .or. y?=w149:bool)
  }
  n229 = call <vilib>:"TCP Listen.vi"("timeout ms (wait forever: -1)"=-1, "port"=u16 5555) -> ("error out"=w4:errorcluster, "connection ID"=w3:refnum<k5>)  [unwired: 5 in, 3 out]
  n230 = while {
    shift-right: [w503] -> w1
    shift-left: w3 -> [w505]
    shift-right: [w502] -> w2
    shift-left: w4 -> [w504]
    i -> [w499]
    stop <- w510 stop-if-true
    n231 = Add(x=w499, y=1) -> (x+y=→"Messages Sent":i32)
    n232 = local read "Trig"() -> (w509:bool)
    n233 = Wait (ms)(milliseconds to wait="Wait [ms]") -> ()  [unwired: 1 out]
    n234 = And(x=w509, y="Transmission") -> (x .and. y?=w507:bool)
    n235 = case shown="True" w507 {
      tunnel: [FALSE TRUE] -> w506
      tunnel: w505 -> [_ w523]
      tunnel: w504 -> [_ w522]
      tunnel: [_ w521] -> w503
      tunnel: [_ w520] -> w502
      frame False {
      }
      frame True {
        n236 = for {
          N: 100 -> [_]
          shift-right: [w527] -> w514
          shift-left: dbl[] [0.0] -> [w528]
          i -> [w526]
          n237 = call "Get_Time.vi"() -> ("double precision float"=w529:dbl)
          n238 = Insert Into Array(array=w528, index=w526, new element=w529) -> (w527:dbl[])
        }
        n239 = local read "Fitted Wavelength (nm) 2"() -> (w515:dbl[][])
        n240 = Insert Into Array(array=w515, index (col)=1, new element=w514) -> (w512:dbl[][])  [unwired: 1 in]
        n241 = Array To Spreadsheet String(array=w512, 3:"%f" ("format string")) -> (spreadsheet string=w518:string)  [unwired: 1 in]
        "String" <- w518
        n242 = String Length(string=w518) -> (length=→"Length":i32)
        n243 = TCP Write(connection ID=w523, data in=w518, error in (no error)=w522) -> (connection ID out=w521:refnum<k5>, error out=w520:errorcluster)  [unwired: 1 in, 1 out]
      }
    }
    "Sending" <- w506
    n244 = local read "Exit"() -> (w510:bool)
  }
  n245 = while {
    tunnel: w18 -> [w530]
    tunnel: [w536] -> w20
    tunnel: [w533] -> w12
    stop <- w532 stop-if-true
    n246 = Get Queue Status(queue=w530) -> (queue out=w537:refnum<queue>, error out=w538:errorcluster, # elements in queue=w535:i32)  [unwired: 2 in, 5 out]
    n247 = Greater Or Equal?(x=w535, y="No. of frames to disc unified") -> (x >= y?=w534:bool)
    n248 = Wait (ms)(milliseconds to wait=u32 100) -> ()  [unwired: 1 out]
    n249 = case shown="True" w534 {
      tunnel: w538 -> [w541 w551]
      tunnel: w537 -> [w540 w552]
      tunnel: [w541 w546] -> w536
      tunnel: [w540 w549] -> w533
      frame False {
      }
      frame True {
        n250 = Flush Queue(queue=w552, error in (no error)=w551) -> (queue out=w549:refnum<queue>, remaining elements=w550:cluster{dbl[][]}[], error out=w547:errorcluster)
        n251 = for {
          tunnel: w550 -> [w556] mode=indexing
          shift-right: [w555] -> w542
          shift-left: dbl[][] [] ("Center pixel") -> [w553]
          n252 = Unbundle(w556) -> (w554:dbl[][])
          n253 = Build Array (concatenate)(w553, w554) -> (w555:dbl[][])
        }
        n254 = local read "refnum out"() -> (w544:refnum<file>)
        n255 = Array To Spreadsheet String(array=w542, 3:"%.5f" ("format string")) -> (spreadsheet string=w545:string)  [unwired: 1 in]
        n256 = Write to Text File(file (use dialog)=w544, text=w545, error in=w547) -> (error out=w546:errorcluster)  [unwired: 1 in, 2 out]
      }
    }
    n257 = local read "Exit"() -> (w532:bool)
  }
  n258 = while {
    tunnel: w18 -> [_]
    tunnel: [w559] -> w17
    stop <- w560 stop-if-true
    n259 = Number To Boolean Array(number="Disc streaming") -> (Boolean array=w561:bool[])
    n260 = Wait (ms)(milliseconds to wait=u32 100) -> ()  [unwired: 1 out]
    n261 = Index Array(array=w561) -> (element=w568:bool)  [unwired: 1 in]
    n262 = Equal?(x="Path", y=path "") -> (x = y?=w567:bool)
    n263 = case shown="False" "Change Disk stream\nfile name" {
      tunnel: w568 -> [w573 _]
      tunnel: w567 -> [w572 _]
      tunnel: "Choose Disk Streaminng file to write" ("prompt") -> [w571 _]
      tunnel: T6."replace or create with confirmation" ("operation (0:open)") -> [w570 w588]
      tunnel: [w569 w587] -> w559
      frame False {
        n264 = case shown="False" w573 {
          tunnel: w570 -> [_ w580]
          tunnel: w571 -> [_ w579]
          tunnel: w572 -> [_ w578]
          tunnel: [errorcluster {"status"=FALSE, "code"=0, "source"=""} ("error out") w577] -> w569
          frame False {
            "Disk streaming enable" <- FALSE ("Disk streaming enable")
          }
          frame True {
            n265 = case shown="True" w578 {
              tunnel: w580 -> [_ w585]
              tunnel: w579 -> [_ w584]
              tunnel: [errorcluster {"status"=FALSE, "code"=0, "source"=""} ("error out") w582] -> w577
              frame False {
              }
              frame True {
                n266 = Open/Create/Replace File(prompt=w584, operation (0:open)=w585) -> (refnum out=w586:refnum<file>, error out=w582:errorcluster)  [unwired: 4 in, 1 out]
                "refnum out" <- w586
                n267 = Refnum to Path(1:w586) -> (0:w583:path)
                n268 = local write "Path"(w583) -> ()
              }
            }
            n269 = local write "Disk streaming enable"(TRUE ("Disk streaming enable")) -> ()
          }
        }
      }
      frame True {
        n270 = local read "refnum out"() -> (w590:refnum<file>)
        n271 = Close File(refnum=w590) -> (error out=w589:errorcluster)  [unwired: 1 in, 1 out]
        n272 = Open/Create/Replace File(error in=w589, operation (0:open)=w588) -> (refnum out=w591:refnum<file>, error out=w587:errorcluster)  [unwired: 4 in, 1 out]
        n273 = local write "refnum out"(w591) -> ()
        n274 = Refnum to Path(1:w591) -> (0:w592:path)
        n275 = local write "Path"(w592) -> ()
      }
    }
    n276 = local read "Exit"() -> (w560:bool)
  }
  n277 = while {
    tunnel: w18 -> [_]
    tunnel: [w602] -> w19
    stop <- w603 stop-if-true
    n278 = local read "Trig"() -> (w601:bool)
    n279 = Or(x="Manuel save\nin datalog file", y="Timed  data log") -> (x .or. y?=w598:bool)
    n280 = Wait (ms)(milliseconds to wait=u32 100) -> ()  [unwired: 1 out]
    n281 = And(x=w598, y=w601) -> (x .and. y?=w597:bool)
    n282 = Or(x=w597, y="Change datalog\nfile name") -> (x .or. y?=w595:bool)
    n283 = case shown="True" w595 {
      tunnel: [errorcluster {"status"=FALSE, "code"=0, "source"=""} ("error out") w610] -> w602
      tunnel: "Timed  data log" -> [_ w609]
      tunnel: "Manuel save\nin datalog file" -> [_ w608]
      tunnel: "Change datalog\nfile name" -> [_ w607]
      frame False {
      }
      frame True {
        n284 = local read "Fitted Wavelength (nm) 2"() -> (w613:dbl[][])
        n285 = local read "Power Array"() -> (w615:dbl[][])
        n286 = Array Size(array=w613) -> (size(s)=w622:i32[])
        n287 = Decrement(x=w622) -> (x-1=w621:i32[])
        n288 = Array Size(array=w615) -> (size(s)=w616:i32[])
        n289 = Decrement(x=w616) -> (x-1=w617:i32[])
        n290 = Index Array(array=w621, index=0) -> (element=w612:i32)
        n291 = Index Array(array=w613, index (row)=w612) -> (element=w619:dbl[])  [unwired: 1 in]
        n292 = local read "Number of pixels"() -> (w606:u16)
        n293 = Index Array(array=w617, index=0) -> (element=w611:i32)
        n294 = Index Array(array=w615, index (row)=w611) -> (element=w614:dbl[])  [unwired: 1 in]
        n295 = call "I_MON_Save_Handling.vi"("Number of pixels"=w606, "Fitted center"=w619, "array"=w614, "Datalog enabled=tru"=w609, "save as"=w607, "Gem 2"=w608) -> ("error out"=w610:errorcluster)  [unwired: 4 in, 1 out]
      }
    }
    n296 = case shown="False" "Change datalog\ntime interval" {
      frame False {
      }
      frame True {
        n297 = global write "D_MON_Global_Save_Handling.vi" "First logdata"(TRUE ("First logdata")) -> ()
      }
    }
    n298 = local read "Exit"() -> (w603:bool)
  }
  n299 = TCP Close Connection(connection ID=w1, error in (no error)=w2) -> ()  [unwired: 1 in, 2 out]
  n300 = local read "refnum out"() -> (w21:refnum<file>)
  n301 = call <vilib>:"Simple Error Handler.vi"("error in (no error)"=w19) -> ()  [unwired: 4 in, 5 out]
  n302 = Close File(refnum=w21, error in=w20) -> ()  [unwired: 2 out]
  n303 = call <vilib>:"Simple Error Handler.vi"("error in (no error)"=w17) -> ()  [unwired: 4 in, 5 out]
  n304 = call <vilib>:"Simple Error Handler.vi"("error in (no error)"=w20) -> ()  [unwired: 4 in, 5 out]
  n305 = call <vilib>:"Simple Error Handler.vi"("error in (no error)"=w23) -> ("error out"=w8:errorcluster)  [unwired: 4 in, 4 out]
  n306 = stacked-sequence {
    tunnel: w8 -> [w624]
    tunnel: [w624] -> w7
    frame #0 {
      n307 = Quit LabVIEW(quit? (T)=TRUE) -> ()
    }
  }
  "error out" <- w7
  n308 = stacked-sequence {
    tunnel: w12 -> [w627]
    tunnel: w23 -> [_]
    tunnel: w10 -> [w625]
    frame #0 {
      n309 = Release Queue(queue=w627) -> (error out=w626:errorcluster)  [unwired: 2 in, 2 out]
      n310 = Release Queue(queue=w625, error in (no error)=w626) -> ()  [unwired: 1 in, 3 out]
    }
  }
